vi "Close.vi"(7 "Abort (F)":bool, 8 "error in (no error)":errorcluster, 11 "Enclave in":refnum<class "Enclave.lvclass">) -> (0 "error out":errorcluster)   [LabVIEW 2022 SP3, in "Enclave.lvlib" / "Enclave.lvclass"]
uses:
  Enclave.lvclass
  Enclave.lvclass/Enclave.ctl
  Writer/Writer.lvclass
  Event/Event.lvclass
  Tag/Tag.lvclass
  Lossless/Lossless.lvclass
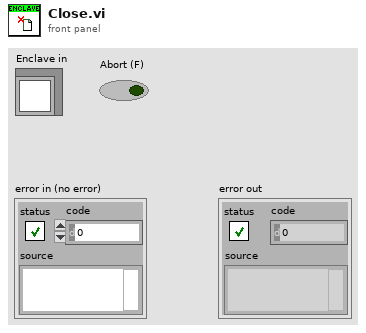
[diagram p1: front panel]
types:
  T1 = typedef "Enclave.lvlib/Enclave.lvclass/Ref Data.ctl" = cluster{"Queues":refnum<class "Lossless.lvclass">[], "Notifiers":refnum<class "Tag.lvclass">[], "Events":refnum<class "Event.lvclass">[], "Writers":refnum<class "Writer.lvclass">[]}
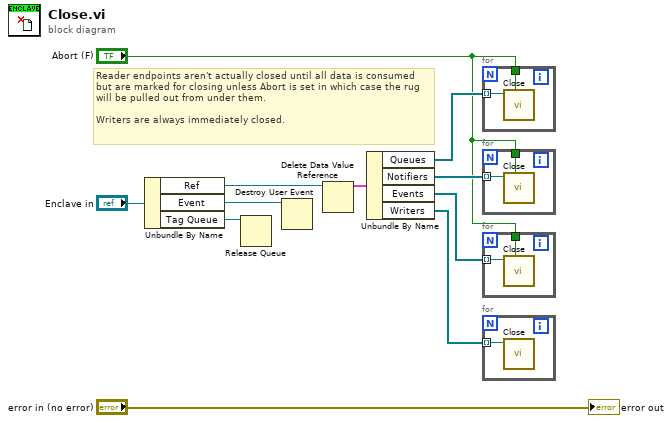
[diagram p0: block diagram]
diagram:
  # "Reader endpoints aren't actually closed until all data is consumed but are marked for closing unless Abort is set in which case the rug will be pulled out from under them.\n\nWriters are always immediately closed."
  n1 = Unbundle By Name("Enclave in") -> ("Ref"=w7:refnum<data-value>, "Event"=w8:refnum<user-event>, "Tag Queue"=w9:refnum<queue>)
  n2 = Release Queue(queue=w9) -> ()  [unwired: 2 in, 3 out]
  n3 = Destroy User Event(user event=w8) -> ()  [unwired: 1 in, 1 out]
  n4 = Delete Data Value Reference(data value reference=w7) -> (data value=w6:T1)  [unwired: 1 in, 1 out]
  n5 = Unbundle By Name(w6) -> ("Queues"=w2:refnum<class "Lossless.lvclass">[], "Notifiers"=w3:refnum<class "Tag.lvclass">[], "Events"=w4:refnum<class "Event.lvclass">[], "Writers"=w5:refnum<class "Writer.lvclass">[])
  n6 = for {
    tunnel: w2 -> [w13] mode=indexing
    tunnel: "Abort (F)" -> [w12]
    n7 = call "Close.vi"("Abort (F)"=w12, "Queue in"=w13) -> ()  [unwired: 9 in, 1 out]
  }
  n8 = for {
    tunnel: w3 -> [w15] mode=indexing
    tunnel: "Abort (F)" -> [w14]
    n9 = call "Close.vi"("Abort (F)"=w14, "Notifier in"=w15) -> ()  [unwired: 9 in, 1 out]
  }
  n10 = for {
    tunnel: w4 -> [w17] mode=indexing
    tunnel: "Abort (F)" -> [w16]
    n11 = call "Close.vi"("Abort (F)"=w16, "Event in"=w17) -> ()  [unwired: 9 in, 1 out]
  }
  n12 = for {
    tunnel: w5 -> [w18] mode=indexing
    n13 = call "Close.vi"("Writer in"=w18) -> ()  [unwired: 10 in, 1 out]
  }
  "error out" <- "error in (no error)"
